vi "BesselI_CDB.vi"(9 "n":i32, 11 "z":cdb format="%#_20g") -> (2 "BesselIn(z)":cdb format="%#_15g")   [LabVIEW 2011]
uses:
  <vilib>/Analysis/2dsp.llb/Integral Method.ctl
  <vilib>/Analysis/1siggen.llb/Ramp Pattern by Samples.vi
  <vilib>/Analysis/NI_AALBase.lvlib
  <vilib>/Analysis/NI_AALPro.lvlib
panel:
  in  "integration method":T1 items=["Trapezoidal Rule", "Simpson's Rule", "Simpson's 3/8 Rule", "Bode Rule"]
  in  "samples":i32=128
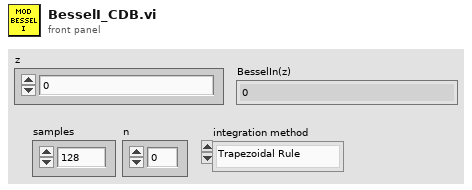
[diagram p1: front panel]
types:
  T1 = typedef "NI_AALPro.lvlib/Integral Method.ctl" = i32
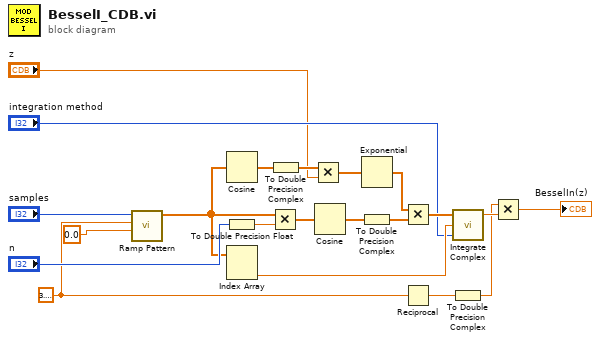
[diagram p0: block diagram]
diagram:
  w2 = 3.141592653589793
  n1 = call-poly <vilib>:"Ramp Pattern.vi"("start"=0.0, "end"=w2, "samples"="samples") -> ("Ramp Pattern"=w9:dbl[])  [unwired: 7 in, 1 out]
  n2 = Cosine(x=w9) -> (cos(x)=w19:dbl[])
  n3 = To Double Precision Float(number="n") -> (double precision float=w16:dbl)
  n4 = Index Array(array=w9) -> (element #2=w8:dbl)  [unwired: 2 in, 1 out]
  n5 = Multiply(x=w9, y=w16) -> (x*y=w15:dbl[])
  n6 = To Double Precision Complex(1:w19) -> (0:w18:cdb[])
  n7 = Multiply(x=w18, y="z") -> (x*y=w14:cdb[])
  n8 = Cosine(x=w15) -> (cos(x)=w13:dbl[])
  n9 = Exponential(1:w14) -> (0:w12:cdb[])
  n10 = To Double Precision Complex(1:w13) -> (0:w11:cdb[])
  n11 = Multiply(x=w12, y=w11) -> (x*y=w10:cdb[])
  n12 = Reciprocal(x=w2) -> (1/x=w5:dbl)
  n13 = call "Integrate Complex.vi"("integration method"="integration method", "dx"=w8, "a+bi"=w10) -> ("int(x) cmplx"=w6:cdb)  [unwired: 2 out]
  n14 = To Double Precision Complex(1:w5) -> (0:w4:cdb)
  n15 = Multiply(x=w4, y=w6) -> (x*y=→"BesselIn(z)":cdb)
